vi "Init Logger.vi"(8 "error in (no error)":errorcluster, 10 "File Send Interval (Seconds)":dbl=600.0) -> (0 "error out":errorcluster, 3 "Logger out.lvclass":refnum<class "Logger.lvclass">)   [LabVIEW 2017, in "Logger.lvclass"]
uses:
  Logger.lvclass
  Logger.lvclass/Logger.ctl
  <vilib>/TagLibrary/Create Tag (String).vi
  <vilib>/TagLibrary/Generate Tag Cluster (String).vi
  <vilib>/TagLibrary/Create Tag (Int).vi
  <vilib>/TagLibrary/Generate Tag Cluster (Int).vi
  <vilib>/Message/Open (Sync).vi
  <vilib>/Message/Subscribe (Sync).vi
  <vilib>/TagLibrary/TagLibrary.lvlib
  <vilib>/Message/Message.lvlib
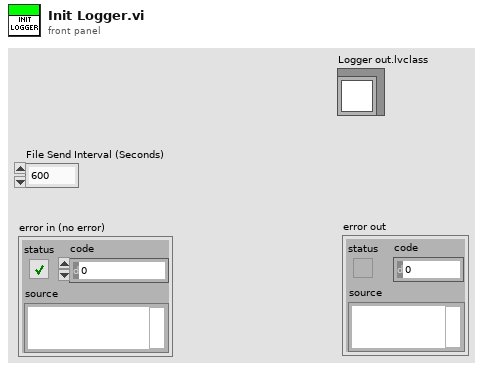
[diagram p1: front panel]
types:
  T1 = cluster{"Tag Reference":refnum<k21>, "Tag Units":string, "Tag Path":string, "Waveform":waveform(dbl), "Log":bool}
  T2 = typedef "TagLibrary.lvlib/TagCluster.ctl" = cluster{"tag reference":refnum<k21>, "value":variant, "timestamp":timestamp, "data type":T3}
  T3 = typedef "TagLibrary.lvlib/DataType.ctl" = enum32{"Double", "Integer", "String"}
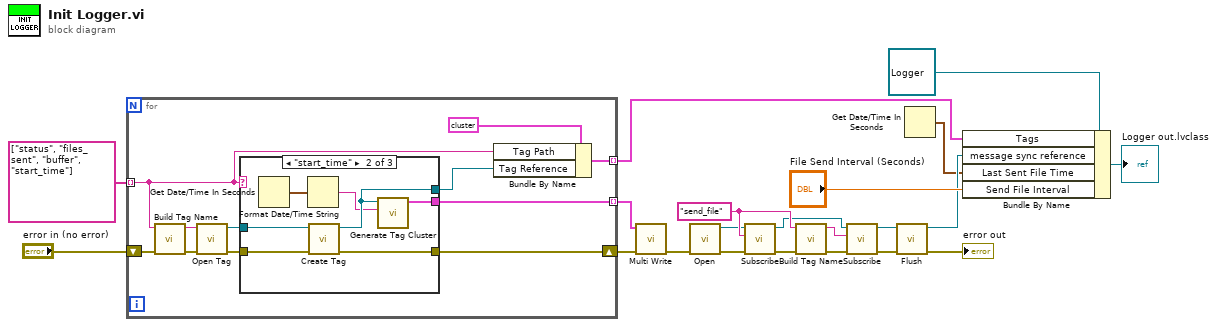
[diagram p0: block diagram]
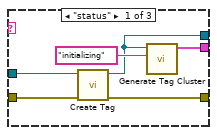
[diagram p2: hidden frame]
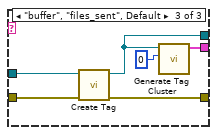
[diagram p3: hidden frame]
diagram:
  w17 = "send_file" ("Tag")
  n1 = for {
    tunnel: [w26] -> w5 mode=indexing
    shift-right: [w27] -> w6
    shift-left: "error in (no error)" -> [w28]
    tunnel: string[] ["status", "files_sent", "buffer", "start_time"] -> [w23] mode=indexing
    tunnel: [w22] -> w3 mode=indexing
    n2 = call "Build Tag Name.vi"("error in (no error)"=w28, "Tag"=w23) -> ("error out"=w29:errorcluster, "System Tag"=w30:string)  [unwired: 8 in]
    n3 = call <vilib>:"Open Tag.vi"("error in (no error)"=w29, "tag path"=w30) -> ("error out"=w31:errorcluster, "tag reference out"=w32:refnum<k21>)  [unwired: 8 in]
    n4 = case shown="\"start_time\"" w23 {
      tunnel: w32 -> [w38 w45 w51]
      tunnel: w31 -> [w37 w44 w50]
      tunnel: [w36 w43 w49] -> w27
      tunnel: [w34 w42 w48] -> w26
      tunnel: [w33 w41 w47] -> w24
      frame "status" {
        n5 = call-poly <vilib>:"Create Tag.vi"("error in (no error)"=w37, "tag reference in"=w38) -> ("error out"=w36:errorcluster, "tag reference out"=w33:refnum<k21>)  [unwired: 8 in]
        n6 = call-poly <vilib>:"Generate Tag Cluster.vi"("string"="initializing", "tag reference in"=w33) -> ("tag cluster"=w34:T2)  [unwired: 9 in]
      }
      frame "start_time" {
        n7 = Get Date/Time In Seconds() -> (seconds since 1Jan1904=w40:timestamp)
        n8 = Format Date/Time String(seconds (now)=w40) -> (date/time string=w39:string)  [unwired: 2 in]
        n9 = call-poly <vilib>:"Create Tag.vi"("error in (no error)"=w44, "tag reference in"=w45) -> ("error out"=w43:errorcluster, "tag reference out"=w41:refnum<k21>)  [unwired: 8 in]
        n10 = call-poly <vilib>:"Generate Tag Cluster.vi"("string"=w39, "tag reference in"=w41) -> ("tag cluster"=w42:T2)  [unwired: 9 in]
      }
      frame "buffer", "files_sent", Default {
        n11 = call-poly <vilib>:"Create Tag.vi"("error in (no error)"=w50, "tag reference in"=w51) -> ("error out"=w49:errorcluster, "tag reference out"=w47:refnum<k21>)  [unwired: 8 in]
        n12 = call-poly <vilib>:"Generate Tag Cluster.vi"("value"=0, "tag reference in"=w47) -> ("tag cluster"=w48:T2)  [unwired: 9 in]
      }
    }
    n13 = Bundle By Name(cluster=T1 {"Tag Reference"="", "Tag Units"="", "Tag Path"="", "Waveform"={"t0"=timestamp(0 s since 1904-01-01), "dt"=1.0, "Y"=[]}, "Log"=FALSE} ("Tag"), "Tag Path"=w23, "Tag Reference"=w24) -> (w22:T1)
  }
  n14 = call <vilib>:"Multi Write.vi"("tag clusters"=w5, "error in (no error)"=w6) -> ("error out"=w8:errorcluster)  [unwired: 7 in, 1 out]
  n15 = call-poly <vilib>:"Open.vi"("error in"=w8) -> ("error out"=w15:errorcluster, "message sync reference"=w16:refnum<k21>)  [unwired: 9 in]
  n16 = call-poly <vilib>:"Subscribe.vi"("error in (no error)"=w15, "topic"=w17, "message sync reference in"=w16) -> ("error out"=w10:errorcluster, "message sync reference out"=w14:refnum<k21>)  [unwired: 7 in]
  n17 = call "Build Tag Name.vi"("error in (no error)"=w10, "Tag"=w17) -> ("error out"=w9:errorcluster, "System Tag"=w18:string)  [unwired: 8 in]
  n18 = call-poly <vilib>:"Subscribe.vi"("error in (no error)"=w9, "topic"=w18, "message sync reference in"=w14) -> ("error out"=w12:errorcluster, "message sync reference out"=w13:refnum<k21>)  [unwired: 7 in]
  n19 = call <vilib>:"Flush.vi"("error in (no error)"=w12, "message sync reference in"=w13) -> ("error out"=→"error out":errorcluster, "message sync reference out"=w11:refnum<k21>)  [unwired: 8 in]
  n20 = Get Date/Time In Seconds() -> (seconds since 1Jan1904=w4:timestamp)
  n21 = Bundle By Name(cluster=refnum<class "Logger.lvclass"> refnum ("Logger out.lvclass"), "Tags"=w3, "message sync reference"=w11, "Last Sent File Time"=w4, "Send File Interval"="File Send Interval (Seconds)") -> (→"Logger out.lvclass":refnum<class "Logger.lvclass">)
